vi "题目6.vi"   [LabVIEW 2017]
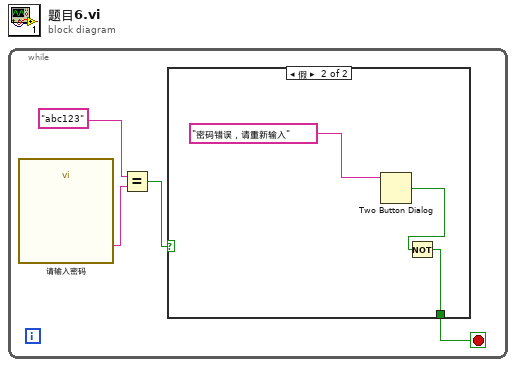
[diagram p0: block diagram]
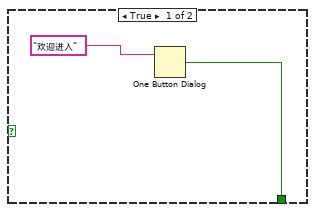
[diagram p2: hidden frame]
diagram:
  n1 = while {
    stop <- w2 stop-if-true
    n2 = call "请输入密码"() -> ("请输入密码"=w3:string)  [unwired: 17 in, 2 out]
    n3 = Equal?(x="abc123", y=w3) -> (x = y?=w4:bool)
    n4 = case shown="假" w4 {
      tunnel: [w5 w7] -> w2
      frame True {
        n5 = One Button Dialog(message="欢迎进入" ("消息")) -> (true=w5:bool)  [unwired: 1 in]
      }
      frame False {
        n6 = Two Button Dialog(message="密码错误，请重新输入" ("消息")) -> (T button?=w8:bool)  [unwired: 2 in]
        n7 = Not(x=w8) -> (.not. x?=w7:bool)
      }
    }
  }
